vi "ReadValByRefString.vi"(0 "Control Ref":refnum<vi>, 2 "Type In":string, 11 "error in":errorcluster caption="entrée d'erreur") -> (4 "Valeur":string, 15 "error out":errorcluster caption="sortie d'erreur")   [LabVIEW 2019]
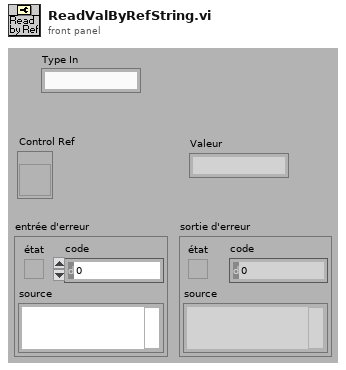
[diagram p1: front panel]
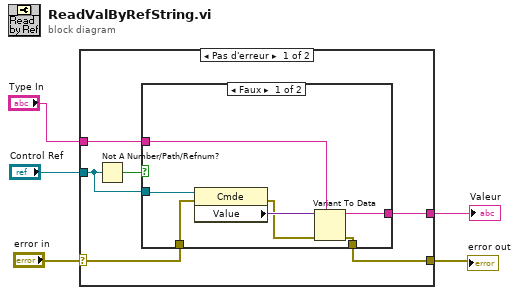
[diagram p0: block diagram]
diagram:
  n1 = case shown="Pas d'erreur" "error in" {
    selector: "error in" -> [w8 w21]
    tunnel: "Control Ref" -> [w10 _]
    tunnel: [w9 _] -> w4
    tunnel: [w7 w21] -> w2
    tunnel: "Type In" -> [w6 _]
    frame No Error {
      n2 = Not A Number/Path/Refnum?(number/path/refnum=w10) -> (NaN/Path/Refnum?=w11:bool)
      n3 = case shown="Faux" w11 {
        tunnel: w10 -> [w18 _]
        tunnel: [w16 w19] -> w9
        tunnel: w8 -> [w13 w20]
        tunnel: [w15 w20] -> w7
        tunnel: w6 -> [w14 w19]
        frame False {
          n4 = property class="Cmde"(reference=w18, error in=w13) -> (error out=w12:errorcluster, "Value"=w17:variant)  [unwired: 1 out]
          n5 = Variant To Data(error in=w12, type=w14, Variant=w17) -> (data=w16:string, error out=w15:errorcluster)
        }
        frame True {
        }
      }
    }
    frame Error {
    }
  }
  "Valeur" <- w4
  "error out" <- w2
